vi "Read.vi"(0 "Task in":refnum<k21>, 1 "Input Rate":dbl, 2 "error in (no error)":errorcluster) -> (3 "Task out":refnum<k21>, 4 "data":dbl[][](array[numeric]), 5 "samples":i32, 6 "error out":errorcluster)   [LabVIEW 2013]
uses:
  <vilib>/DAQmx/read.llb/DAQmx Read (Analog 2D DBL NChan NSamp).vi
  <vilib>/DAQmx/configure/timing.llb/DAQmx Timing (Sample Clock).vi
  <vilib>/DAQmx/miscellaneous.llb/DAQmx Fill In Error Info.vi
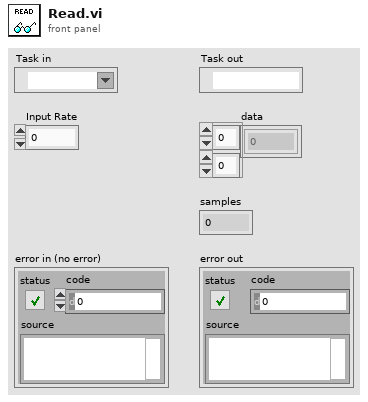
[diagram p1: front panel]
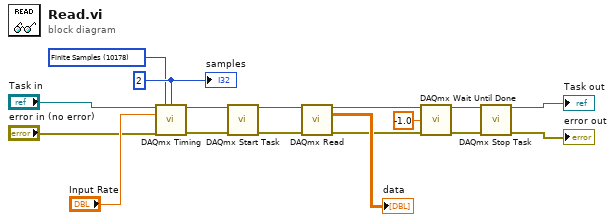
[diagram p0: block diagram]
diagram:
  w17 = 2 ("samples per channel")
  w4 = 10178 items=["Finite Samples"=10178, "Continuous Samples"=10123, "Hardware Timed Single Point"=12522] ("sample mode")
  n1 = call-poly <vilib>:"DAQmx Timing.vi"("task/channels in"="Task in", "sample mode"=w4, "samples per channel"=w17, "rate"="Input Rate", "error in"="error in (no error)") -> ("task out"=w5:refnum<k21>, "error out"=w6:errorcluster)  [unwired: 9 in]
  n2 = call <vilib>:"DAQmx Start Task.vi"("task/channels in"=w5, "error in"=w6) -> ("task out"=w7:refnum<k21>, "error out"=w8:errorcluster)  [unwired: 12 in]
  n3 = call-poly <vilib>:"DAQmx Read.vi"("task/channels in"=w7, "error in"=w8) -> ("task out"=w9:refnum<k21>, "data"=→"data":dbl[][], "error out"=w10:errorcluster)  [unwired: 11 in]
  n4 = call <vilib>:"DAQmx Wait Until Done.vi"("task/channels in"=w9, "timeout (sec)"=-1.0, "error in"=w10) -> ("task out"=w12:refnum<k21>, "error out"=w13:errorcluster)  [unwired: 11 in]
  n5 = call <vilib>:"DAQmx Stop Task.vi"("task/channels in"=w12, "error in"=w13) -> ("task out"=→"Task out":refnum<k21>, "error out"=→"error out":errorcluster)  [unwired: 12 in]
  "samples" <- w17
